vi "FSW_Renamed Event Callback.vi"(4 "FileEvent":refnum<user-event>, 5 "事件数据":cluster{"sender":refnum<k24>, "e":refnum<k24>}, 6 "控件引用":refnum<k24>, 7 "事件通用数据":cluster{"事件源":i32, "事件类型":u32, "时间标识":u32}) -> ()   [LabVIEW 2013]
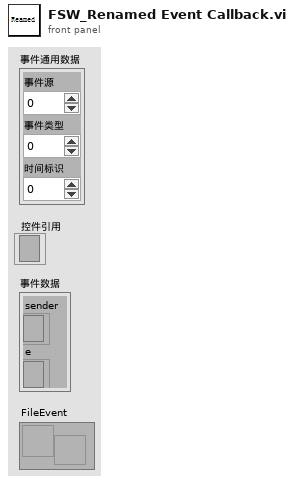
[diagram p1: front panel]
types:
  T1 = cluster{"ChangeType":i32, "FullPath":string, "Name":string, "OldFullPath":string, "OldName":string}
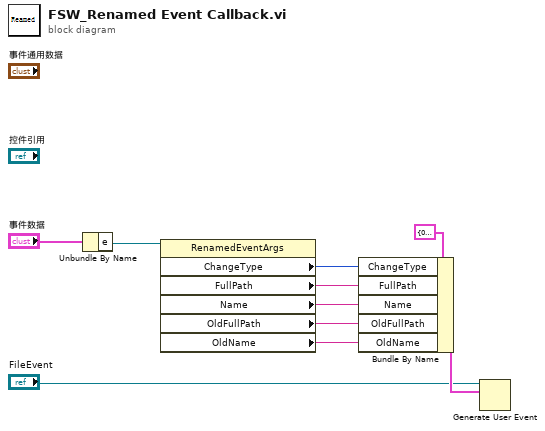
[diagram p0: block diagram]
diagram:
  n1 = Unbundle By Name("事件数据") -> ("e"=w10:refnum<k24>)
  n2 = property on="属性节点" class="RenamedEventArgs"(reference=w10) -> ("ChangeType"=w7:i32, "FullPath"=w6:string, "Name"=w5:string, "OldFullPath"=w2:string, "OldName"=w1:string)  [unwired: 1 in, 2 out]
  n3 = Bundle By Name(cluster=T1 {"ChangeType"=0, "FullPath"="", "Name"="", "OldFullPath"="", "OldName"=""} ("事件数据"), "ChangeType"=w7, "FullPath"=w6, "Name"=w5, "OldFullPath"=w2, "OldName"=w1) -> (w8:T1)
  n4 = Generate User Event(user event="FileEvent", event data cluster=w8) -> ()  [unwired: 2 in, 2 out]
